vi "Get Created Attributes.vi"(10 "Alias":string, 11 "Base Actor in":refnum<class "Base Actor.lvclass">) -> (1 "Is Found":bool, 2 "Created Attributes":refnum<class "Attributes.lvclass">)   [LabVIEW 2020, in "jettl.lvlib" / "Actor.lvlib" / "Base Actor.lvclass"]
uses:
  Base Actor.lvclass
  Attributes/Attributes/Attributes.lvclass
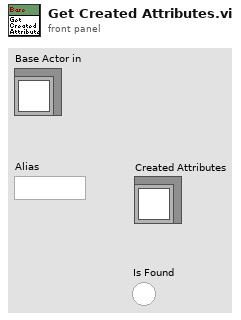
[diagram p1: front panel]
types:
  T1 = typedef "jettl.lvlib/Actor.lvlib/Base Actor.lvclass/Map of Created Attributes.ctl" = map{string, refnum<class "Attributes.lvclass">}
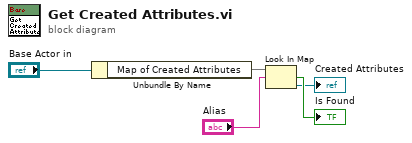
[diagram p0: block diagram]
diagram:
  n1 = Unbundle By Name("Base Actor in") -> ("Map of Created Attributes"=w4:T1)
  n2 = Look In Map(map=w4, key="Alias") -> (key not found?=→"Is Found":bool, value=→"Created Attributes":refnum<class "Attributes.lvclass">)  [unwired: 1 in]
